vi "rampage.vi"() -> ()   [LabVIEW 2010, in "Rampage.lvrbt"]
uses:
  Rampage.lvrbt
  <vilib>/NXT/Subs/MotorOutput.ctl
  <vilib>/NXT/NXTIO Xnodes/AddressXNode/NXTIOAddress.xnode
  <vilib>/NXT/Subs/MotorXNode.DC Motor Type.ctl
  <vilib>/NXT/Subs/MotorXNode.1DCMotor.ctl
  <vilib>/NXT/Subs/LVHSConnector.ctl
  <vilib>/NXT/Subs/MotorXNode.2DCMotor.ctl
  <vilib>/NXT/NXTIO Xnodes/NXTIOXNode/NXTIO.xnode
  <vilib>/FTC/FTC Interpret Motor Power From Left Y Axis.vi
  <vilib>/NXT/Dual Mode Library/prims/inRangeAndCoerce/inRangeAndCoerce_int.vi
  <vilib>/NXT/Dual Mode Library/Motors/MotorOn.vi
  <vilib>/FTC/FTC Interpret Motor Power From Right Y Axis.vi
  <vilib>/NXT/NXTIO Xnodes/NXTIONodeSubVIs/TETRIX IO Stop DC Motors.vi
  <vilib>/NXT/NXTIO Xnodes/NXTIONodeSubVIs/TETRIX IO Move DC Motors.vi
  <vilib>/FTC/FTC Calculate Drive Power - Tank.vi
  <vilib>/NXT/Dual Mode Library/Motors/oldLightOn.vi
  <vilib>/NXT/Dual Mode Library/Motors/oldLightOff.vi
panel:
  in  "Drive Power":i32=100
  in  "Elbow\n Position":i32
  # "This VI was generated based on your configuration in the Remote Control Editor. You may modify the code as needed for your robot. To test this program for an FTC match, return to the Remote Control Editor, select the \"Run Program\" tab, and choose \"FTC Game\"."
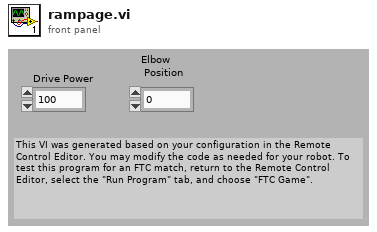
[diagram p1: front panel]
types:
  T1 = typedef "LVHSConnector.ctl" = cluster{"Hardware":string, "Flattened String":string}
  T2 = typedef "FTC ControllerState.ctl" = cluster{"Left X":i8, "Left Y":i8, "Right X":i8, "Right Y":i8, "Button Encoding 9-12":u8, "Button Encoding 1-8":u8, "POV":T3}
  T3 = typedef "FTC POVState.ctl" = i8
  T4 = typedef "FTC ButtonEventType.ctl" = enum16{"Pressed", "Released"}
  T5 = cluster{"Button ID":enum16{"None", "Button 1", "Button 2", "Button 3", "Button 4", "Button 5", "Button 6", "Button 7", "Button 8", "Button 9", "Button 10", "Button 11", "Button 12", "POV Up", "POV Up Right", "POV Right", "POV Down Right", "POV Down", "POV Down Left", "POV Left", "POV Up Left"}, "Event Type":T4}[]
  T6 = enum16{"None", "Button 1", "Button 2", "Button 3", "Button 4", "Button 5", "Button 6", "Button 7", "Button 8", "Button 9", "Button 10", "Button 11", "Button 12", "POV Up", "POV Up Right", "POV Right", "POV Down Right", "POV Down", "POV Down Left", "POV Left", "POV Up Left"}
  T7 = typedef "MotorOutput.ctl" = u8
  T8 = typedef "MotorXNode.DC Motor Type.ctl" = enum16{"DC Motor"}
  T9 = cluster{"DC Motor":T8, "Address":i16, "Address":i16}
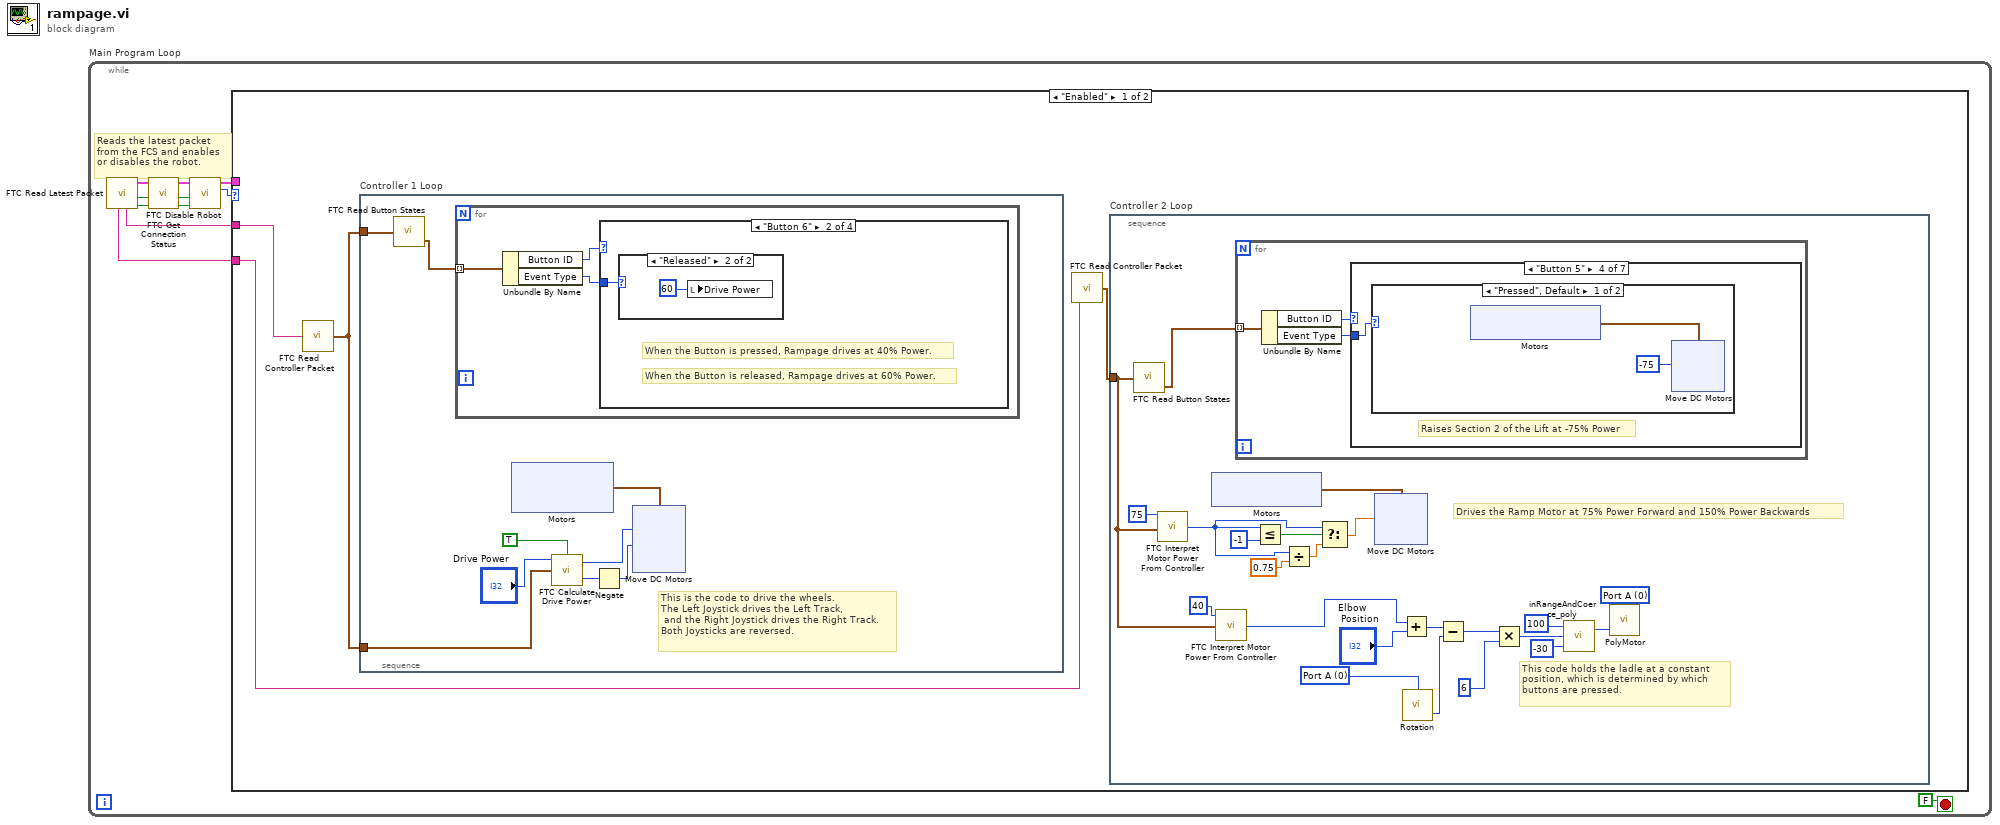
[diagram p0: block diagram]
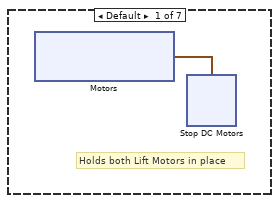
[diagram p2: hidden frame]
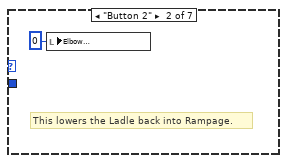
[diagram p3: hidden frame]
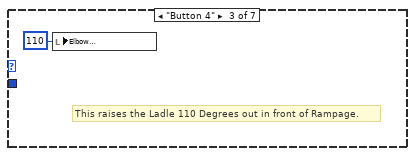
[diagram p4: hidden frame]
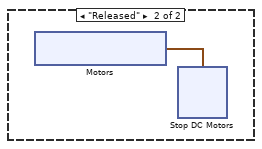
[diagram p5: hidden frame]
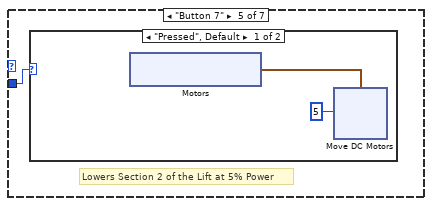
[diagram p6: hidden frame]
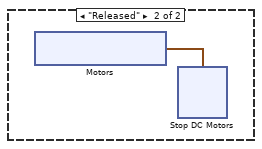
[diagram p7: hidden frame]
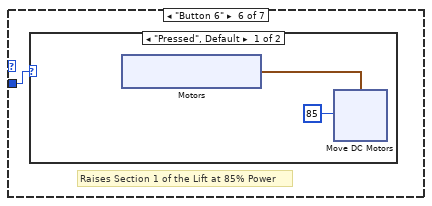
[diagram p8: hidden frame]
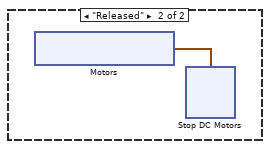
[diagram p9: hidden frame]
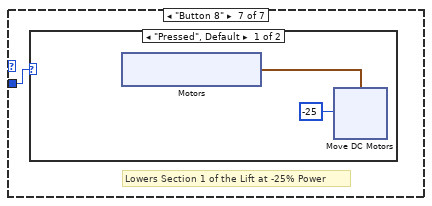
[diagram p10: hidden frame]
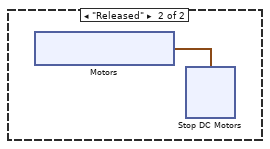
[diagram p11: hidden frame]
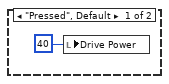
[diagram p13: hidden frame]
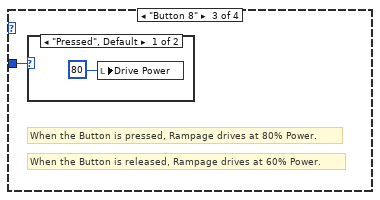
[diagram p14: hidden frame]
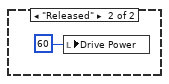
[diagram p15: hidden frame]
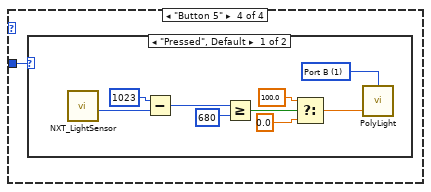
[diagram p16: hidden frame]
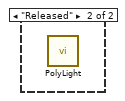
[diagram p17: hidden frame]
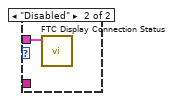
[diagram p18: hidden frame]
diagram:
  n1 = while "Main Program Loop" {
    stop <- FALSE stop-if-true
    # "Reads the latest packet\nfrom the FCS and enables\nor disables the robot."
    n2 = call <vilib>:"FTC Read Latest Packet.vi"() -> ("Packet Received?"=w8:bool, "Stopped?"=w5:bool, "NXT"=w7:T1, "Controller 1"=w10:string, "Controller 2"=w9:string)  [unwired: 6 in, 1 out]
    n3 = call <vilib>:"FTC Get Connection Status.vi"("Packet Received?"=w8, "Stopped?"=w5, "NXT"=w7) -> ("Online?"=w2:bool, "Stopped?"=w3:bool, "NXT"=w4:T1)  [unwired: 5 in]
    n4 = call <vilib>:"FTC Disable Robot.vi"("Online?"=w2, "Stopped?"=w3, "NXT"=w4) -> ("Enabled?"=w6:enum16{"Disabled", "Enabled"}, "NXT"=w1:T1)  [unwired: 3 in]
    n5 = case "disableCase" shown="\"Enabled\"" w6 {
      tunnel: w10 -> [w15 _]
      tunnel: w9 -> [w12 _]
      tunnel: w1 -> [_ w181]
      frame "Enabled" {
        n6 = call <vilib>:"FTC Read Controller Packet.vi"("Packet"=w15) -> ("Controller State"=w13:T2)  [unwired: 4 in]
        n7 = stacked-sequence "Controller 1 Loop" {
          tunnel: w13 -> [w150]
          tunnel: w13 -> [w146]
          frame #0 {
            # "This is the code to drive the wheels.\nThe Left Joystick drives the Left Track,\n and the Right Joystick drives the Right Track.\nBoth Joysticks are reversed."
            n8 = call <vilib>:"FTC Read Button States.vi"("Controller State"=w146) -> ("Button Events"=w145:T5)  [unwired: 2 in, 1 out]
            n9 = for {
              tunnel: w145 -> [w153] mode=indexing
              n10 = Unbundle By Name(w153) -> ("Button ID"=w152:T6, "Event Type"=w151:T4)
              n11 = case shown="\"Button 6\"" w152 {
                tunnel: w151 -> [_ w154 w157 w160]
                frame "None", Default {
                }
                frame "Button 6" {
                  # "When the Button is released, Rampage drives at 60% Power."
                  # "When the Button is pressed, Rampage drives at 40% Power."
                  n12 = case shown="\"Released\"" w154 {
                    frame "Pressed", Default {
                      n13 = local write "Drive Power"(40 ("Drive Power")) -> ()
                    }
                    frame "Released" {
                      n14 = local write "Drive Power"(60 ("Drive Power")) -> ()
                    }
                  }
                }
                frame "Button 8" {
                  # "When the Button is released, Rampage drives at 60% Power."
                  # "When the Button is pressed, Rampage drives at 80% Power."
                  n15 = case shown="\"Pressed\", Default" w157 {
                    frame "Pressed", Default {
                      n16 = local write "Drive Power"(80 ("Drive Power")) -> ()
                    }
                    frame "Released" {
                      n17 = local write "Drive Power"(60 ("Drive Power")) -> ()
                    }
                  }
                }
                frame "Button 5" {
                  n18 = case shown="\"Pressed\", Default" w160 {
                    frame "Pressed", Default {
                      w166 = T7 1 items=["Port A"=0, "Port B"=1, "Port C"=2, "Ports A & B"=4, "Ports A & C"=5, "Ports B & C"=6, "All Ports"=3] ("Output Port (All Ports)")
                      n19 = call <vilib>:"NXT_LightSensor.vi"() -> ("Raw Value"=w167:u16)  [unwired: 8 in, 3 out]
                      n20 = Subtract(x=u16 1023, y=w167) -> (x-y=w169:u16)
                      n21 = Greater Or Equal?(x=w169, y=i16 680) -> (x >= y?=w162:bool)
                      n22 = Select(t=100.0, s=w162, f=0.0) -> (s? t:f=w165:dbl)
                      n23 = call-poly <vilib>:"PolyLight.vi"("Power (75)"=w165, "Output Port (All Ports)"=w166) -> ()  [unwired: 2 in, 1 out]
                    }
                    frame "Released" {
                      n24 = call-poly <vilib>:"PolyLight.vi"() -> ()  [unwired: 4 in, 1 out]
                    }
                  }
                }
              }
            }
            n25 = xnode ("Motors")() -> ("DC Motor"=w148:T9)
            n26 = call-poly <vilib>:"FTC Calculate Drive Power.vi"("Reverse"=TRUE, "Controller State"=w150, "Power Level (50)"="Drive Power") -> ("Right Motor Power"=w143:i8, "Left Motor Power"=w147:i8)  [unwired: 1 in]
            n27 = Negate(x=w143) -> (-x=w142:i8)
            n28 = xnode ("Move DC Motors")("Power/Speed 2"=w142, "Power/Speed 1"=w147, "Motors"=w148) -> ()  [unwired: 1 in, 1 out]
          }
        }
        n29 = call <vilib>:"FTC Read Controller Packet.vi"("Packet"=w12) -> ("Controller State"=w14:T2)  [unwired: 4 in]
        n30 = stacked-sequence "Controller 2 Loop" {
          tunnel: w14 -> [w30]
          frame #0 {
            w35 = T7 0 items=["Port A"=0, "Port B"=1, "Port C"=2, "Ports A & B"=4, "Ports A & C"=5, "Ports B & C"=6, "All Ports"=3] ("Output Port (All Ports)")
            w32 = u8 0 items=["Port A", "Port B", "Port C"] ("Port (Port A)")
            # "Drives the Ramp Motor at 75% Power Forward and 150% Power Backwards"
            # "This code holds the ladle at a constant \nposition, which is determined by which \nbuttons are pressed."
            n31 = call <vilib>:"FTC Read Button States.vi"("Controller State"=w30) -> ("Button Events"=w38:T5)  [unwired: 2 in, 1 out]
            n32 = call-poly <vilib>:"FTC Interpret Motor Power From Controller.vi"("Controller State"=w30, "Power Level (50)"=i8 75) -> ("Power"=w16:i8)  [unwired: 1 in]
            n33 = xnode "Motors"() -> ("DC Motor"=w36:cluster{"DC Motor":T8, "Address":i16})
            n34 = call-poly <vilib>:"FTC Interpret Motor Power From Controller.vi"("Controller State"=w30, "Power Level (50)"=i8 40) -> ("Power"=w29:i8)  [unwired: 1 in]
            n35 = for "buttonAction" {
              tunnel: w38 -> [w49] mode=indexing
              n36 = Unbundle By Name(w49) -> ("Button ID"=w48:T6, "Event Type"=w50:T4)
              n37 = case "EventCase2" shown="\"Button 5\"" w48 {
                tunnel: w50 -> [_ _ _ w62 w82 w102 w122]
                frame Default {
                  # "Holds both Lift Motors in place"
                  n38 = xnode "Motors"() -> ("DC Motor"=w51:T9)
                  n39 = xnode "Stop DC Motors"("Motors"=w51) -> ()  [unwired: 1 in, 1 out]
                }
                frame "Button 2" {
                  # "This lowers the Ladle back into Rampage."
                  n40 = local write "Elbow\n Position"(0 ("Button 1")) -> ()
                }
                frame "Button 4" {
                  # "This raises the Ladle 110 Degrees out in front of Rampage."
                  n41 = local write "Elbow\n Position"(110 ("Button 1")) -> ()
                }
                frame "Button 5" {
                  # "Raises Section 2 of the Lift at -75% Power"
                  n42 = case shown="\"Pressed\", Default" w62 {
                    frame "Pressed", Default {
                      n43 = xnode "Motors"() -> ("DC Motor"=w64:cluster{"DC Motor":T8, "Address":i16})
                      n44 = xnode "Move DC Motors"("Power/Speed 1"=i8 -75, "Motors"=w64) -> ()  [unwired: 1 in, 1 out]
                    }
                    frame "Released" {
                      n45 = xnode "Motors"() -> ("DC Motor"=w74:cluster{"DC Motor":T8, "Address":i16})
                      n46 = xnode "Stop DC Motors"("Motors"=w74) -> ()  [unwired: 1 in, 1 out]
                    }
                  }
                }
                frame "Button 7" {
                  # "Lowers Section 2 of the Lift at 5% Power"
                  n47 = case shown="\"Pressed\", Default" w82 {
                    frame "Pressed", Default {
                      n48 = xnode "Motors"() -> ("DC Motor"=w84:cluster{"DC Motor":T8, "Address":i16})
                      n49 = xnode "Move DC Motors"("Power/Speed 1"=i8 5, "Motors"=w84) -> ()  [unwired: 1 in, 1 out]
                    }
                    frame "Released" {
                      n50 = xnode "Motors"() -> ("DC Motor"=w94:cluster{"DC Motor":T8, "Address":i16})
                      n51 = xnode "Stop DC Motors"("Motors"=w94) -> ()  [unwired: 1 in, 1 out]
                    }
                  }
                }
                frame "Button 6" {
                  # "Raises Section 1 of the Lift at 85% Power"
                  n52 = case shown="\"Pressed\", Default" w102 {
                    frame "Pressed", Default {
                      n53 = xnode "Motors"() -> ("DC Motor"=w104:cluster{"DC Motor":T8, "Address":i16})
                      n54 = xnode "Move DC Motors"("Power/Speed 1"=i8 85, "Motors"=w104) -> ()  [unwired: 1 in, 1 out]
                    }
                    frame "Released" {
                      n55 = xnode "Motors"() -> ("DC Motor"=w114:cluster{"DC Motor":T8, "Address":i16})
                      n56 = xnode "Stop DC Motors"("Motors"=w114) -> ()  [unwired: 1 in, 1 out]
                    }
                  }
                }
                frame "Button 8" {
                  # "Lowers Section 1 of the Lift at -25% Power"
                  n57 = case shown="\"Pressed\", Default" w122 {
                    frame "Pressed", Default {
                      n58 = xnode "Motors"() -> ("DC Motor"=w124:cluster{"DC Motor":T8, "Address":i16})
                      n59 = xnode "Move DC Motors"("Power/Speed 1"=i8 -25, "Motors"=w124) -> ()  [unwired: 1 in, 1 out]
                    }
                    frame "Released" {
                      n60 = xnode "Motors"() -> ("DC Motor"=w134:cluster{"DC Motor":T8, "Address":i16})
                      n61 = xnode "Stop DC Motors"("Motors"=w134) -> ()  [unwired: 1 in, 1 out]
                    }
                  }
                }
              }
            }
            n62 = Less Or Equal?(x=w16, y=i8 -1) -> (x <= y?=w20:bool)
            n63 = Divide(x=w16, y=0.75) -> (x/y=w18:dbl)
            n64 = Select(t=w16, s=w20, f=w18) -> (s? t:f=w19:dbl)
            n65 = xnode "Move DC Motors"("Power/Speed 1"=w19, "Motors"=w36) -> ()  [unwired: 1 in, 1 out]
            n66 = Add(x=w29, y="Elbow\n Position") -> (x+y=w27:i32)
            n67 = call <vilib>:"Rotation.vi"("Port (Port A)"=w32) -> ("Angle of Rotation"=w33:i32)  [unwired: 2 in, 1 out]
            n68 = Subtract(x=w27, y=w33) -> (x-y=w34:i32)
            n69 = Multiply(x=w34, y=6) -> (x*y=w26:i32)
            n70 = call-poly <vilib>:"inRangeAndCoerce_poly.vi"("lower limit"=-30, "x"=w26, "upper limit"=100) -> ("coerced(x)"=w23:i32)  [unwired: 1 out]
            n71 = call-poly <vilib>:"PolyMotor.vi"("Power (75)"=w23, "Output Port (All Ports)"=w35) -> ()  [unwired: 2 in, 1 out]
          }
        }
      }
      frame "Disabled" {
        n72 = call <vilib>:"FTC Display Connection Status.vi"("NXT"=w181) -> ()  [unwired: 10 in, 1 out]
      }
    }
  }
